vi "Asylum_Driver_Lithography_Convert_Units.vi"(6 "Amplifier":dbl=20.0 format="%#_13g", 8 "error in (no error)":errorcluster, 11 "Lithography Data":T2(array[cluster])) -> (0 "error out":errorcluster, 3 "Lithography Data":T2(array[cluster]))   [LabVIEW 2020]
uses:
  <userlib>/LevyLab/Relay Box/Type_defs/Resistor--enum.ctl
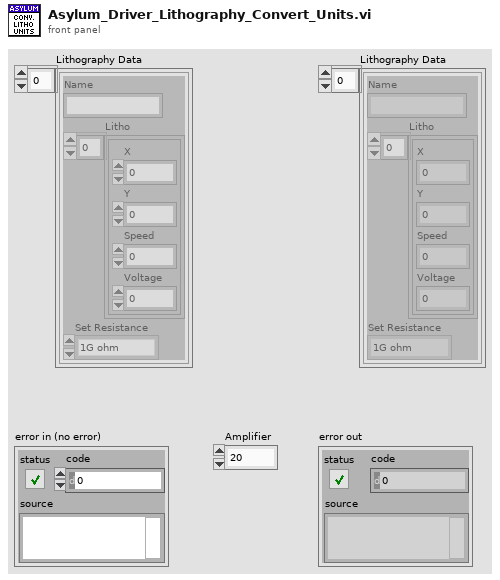
[diagram p1: front panel]
types:
  T1 = typedef "Resistor--enum.ctl" = enum16{"open", "discharge tip", "0 ohms", "100k ohm", "10M ohm", "1G ohm"}
  T2 = cluster{"Name":string, "Litho":cluster{"X":dbl, "Y":dbl, "Speed":dbl, "Voltage":dbl}[], "Set Resistance":T1}[]
  T3 = cluster{"X":dbl, "Y":dbl, "Speed":dbl, "Voltage":dbl}[]
  T4 = cluster{"X":dbl, "Y":dbl, "Speed":dbl, "Voltage":dbl}
  T5 = cluster{"Name":string, "Litho":cluster{"X":dbl, "Y":dbl, "Speed":dbl, "Voltage":dbl}[], "Set Resistance":T1}
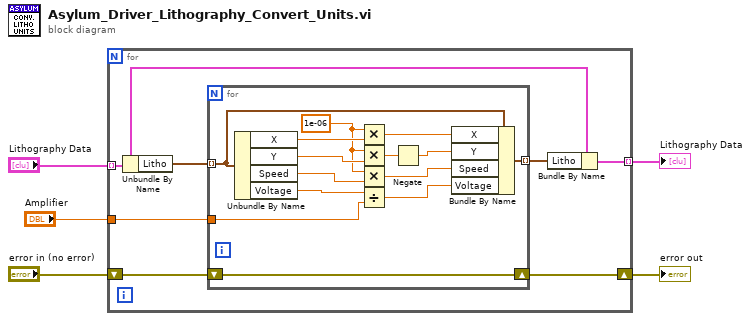
[diagram p0: block diagram]
diagram:
  n1 = for {
    tunnel: "Lithography Data" -> [w12] mode=indexing
    tunnel: [w9] -> w4 mode=indexing
    shift-right: [w8] -> w3
    shift-left: "error in (no error)" -> [w7]
    tunnel: "Amplifier" -> [w6]
    n2 = Unbundle By Name(w12) -> ("Litho"=w11:T3)
    n3 = for {
      tunnel: w11 -> [w26] mode=indexing
      tunnel: [w16] -> w10 mode=indexing
      shift-right: [w15] -> w8
      shift-left: w7 -> [w15]
      tunnel: w6 -> [w13]
      w17 = 1e-06
      n4 = Unbundle By Name(w26) -> ("X"=w18:dbl, "Y"=w19:dbl, "Speed"=w20:dbl, "Voltage"=w21:dbl)
      n5 = Multiply(x=w17, y=w18) -> (x*y=w25:dbl)
      n6 = Multiply(x=w17, y=w19) -> (x*y=w24:dbl)
      n7 = Multiply(x=w17, y=w20) -> (x*y=w23:dbl)
      n8 = Divide(x=w21, y=w13) -> (x/y=w22:dbl)
      n9 = Negate(x=w24) -> (-x=w14:dbl)
      n10 = Bundle By Name(cluster=w26, "X"=w25, "Y"=w14, "Speed"=w23, "Voltage"=w22) -> (w16:T4)
    }
    n11 = Bundle By Name(cluster=w12, "Litho"=w10) -> (w9:T5)
  }
  "Lithography Data" <- w4
  "error out" <- w3
